vi "G3 Get LV Class Default Value.vi"(0 "Export Type":path, 5 "Component Definition ini Path":path, 11 "error in (no error)":errorcluster) -> (4 "LabVIEW Object out":refnum<class>, 15 "error out":errorcluster)   [LabVIEW 2017, in "CL_G3_VIComponentBuilder.lvlib"]
uses:
  CL_G3_VIComponentBuilder.lvlib
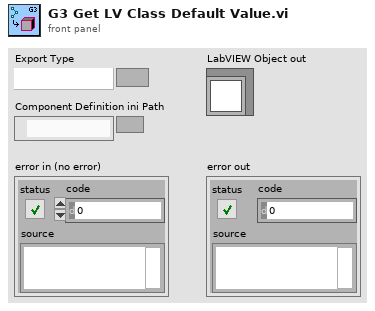
[diagram p1: front panel]
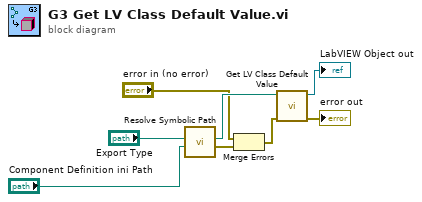
[diagram p0: block diagram]
diagram:
  n1 = call "Resolve Symbolic Path.vi"("Component Root Path"="Component Definition ini Path", "Path In"="Export Type") -> ("error out"=w1:errorcluster, "Path Out"=w7:path)  [unwired: 8 in]
  n2 = Merge Errors("error in (no error)", w1) -> (w2:errorcluster)
  n3 = call <vilib>:"Get LV Class Default Value.vi"("error in (no error)"=w2, "class path"=w7) -> ("error out"=→"error out":errorcluster, "object"=→"LabVIEW Object out":refnum<class>)  [unwired: 8 in]
